vi "Test Trigger VI.vi"() -> ()   [LabVIEW 2011]
uses:
  <vilib>/Utility/file.llb/Write To Spreadsheet File (DBL).vi
panel:
  out "Channel 3 Mean":dbl=1.0
  out "Channel 3 Buffer":dbl[](array[numeric])
  in  "file path (use dialog)":path
  out "V1 Buffer":dbl[](array[numeric]) format="%#_10g"
  out "V1/V2 Buffer":dbl[](array[numeric]) format="%#_10g"
  out "V2 Mean":dbl
  in  "milliseconds to wait":u32=2500
  out "Ratio V1/V2 Mean":dbl=1.0
  out "Shots Measured":ext[][](array[numeric]) format="%#_10g"
  out "V1 Mean":dbl=1.0
  in  "Shots":i32
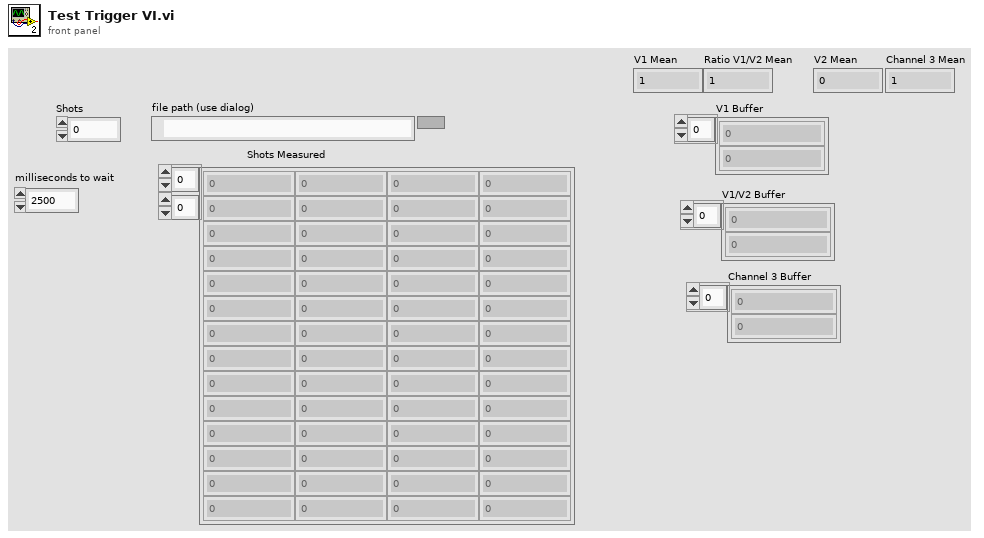
[diagram p1: front panel]
types:
  T1 = enum16{"open", "replace", "create", "open or create", "replace or create", "replace or create with confirmation"}
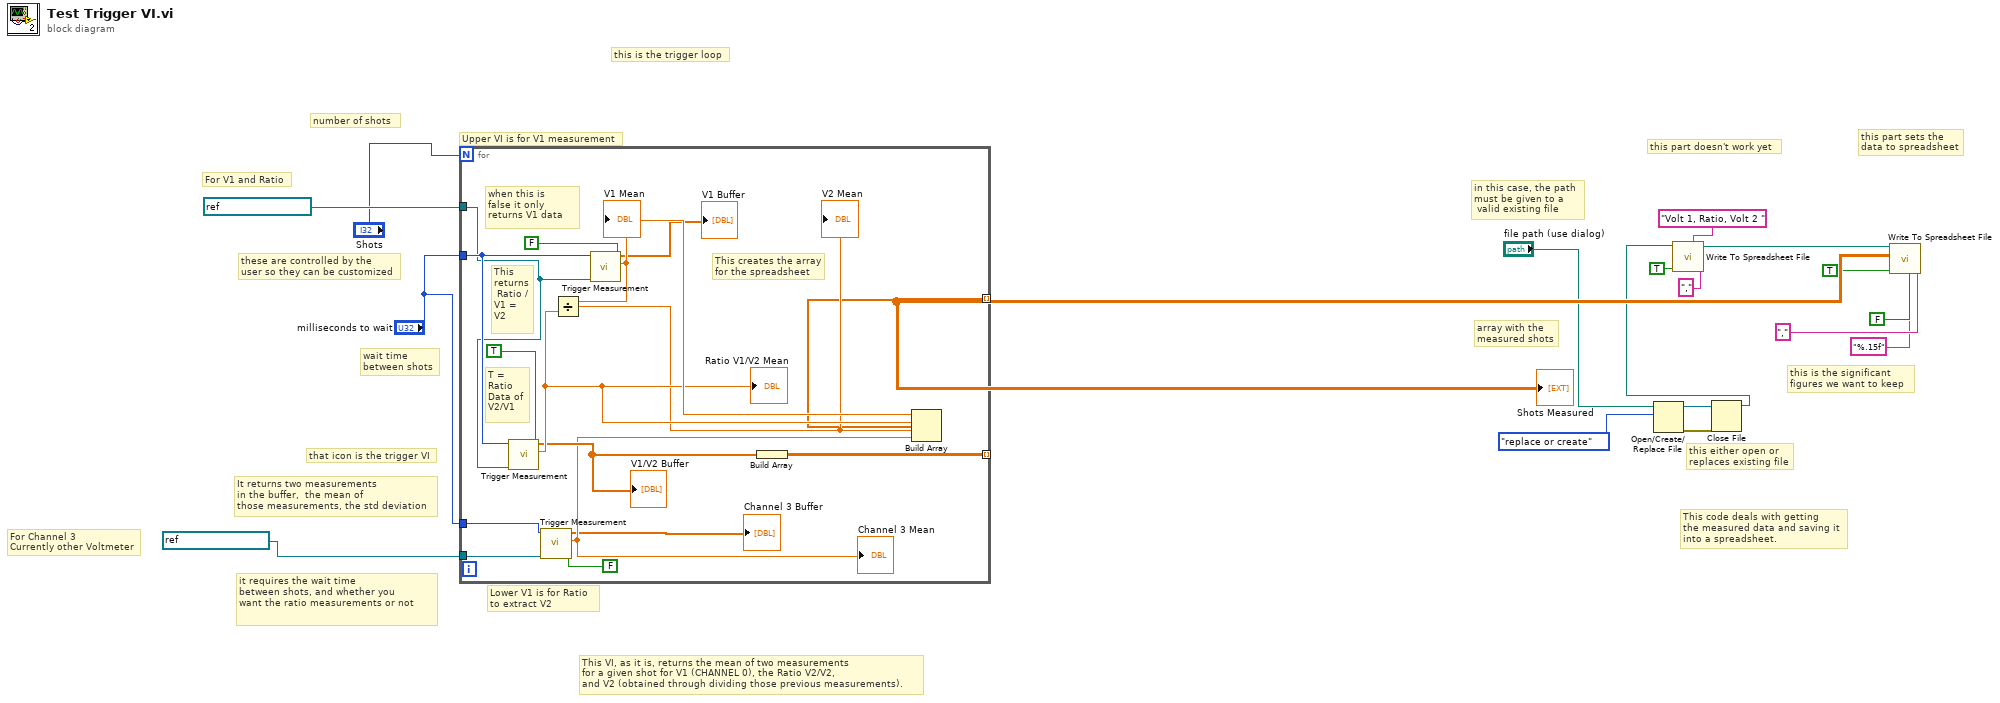
[diagram p0: block diagram]
diagram:
  # "For Channel 3\nCurrently other Voltmeter"
  # "For V1 and Ratio"
  # "This code deals with getting\nthe measured data and saving it\ninto a spreadsheet."
  # "Lower V1 is for Ratio \nto extract V2"
  # "Upper VI is for V1 measurement"
  # "This VI, as it is, returns the mean of two measurements\nfor a given shot for V1 (CHANNEL 0), the Ratio V2/V2, \nand V2 (obtained through dividing those previous measurements)."
  # "it requires the wait time \nbetween shots, and whether you \nwant the ratio measurements or not"
  # "It returns two measurements \nin the buffer,  the mean of \nthose measurements, the std deviation"
  # "that icon is the trigger VI"
  # "this is the trigger loop"
  # "these are controlled by the \nuser so they can be customized"
  # "number of shots"
  # "wait time \nbetween shots"
  # "this is the significant \nfigures we want to keep"
  # "this either open or \nreplaces existing file"
  # "array with the\nmeasured shots"
  # "in this case, the path \nmust be given to a\n valid existing file"
  # "this part sets the \ndata to spreadsheet"
  # "this part doesn't work yet"
  n1 = for {
    N: "Shots" -> [_]
    tunnel: [w27] -> w18 mode=indexing
    tunnel: "milliseconds to wait" -> [w29]
    tunnel: [w25] -> _ mode=indexing
    tunnel: refnum<visa-resource-name> "GPIB0::7::INSTR" ("VISA resource name") -> [w24]
    tunnel: refnum<visa-resource-name> "GPIB0::5::INSTR" ("VISA resource name") -> [w23]
    tunnel: "milliseconds to wait" -> [w22]
    # "This creates the array \nfor the spreadsheet"
    # "T =\nRatio Data of\nV2/V1"
    # "This returns\n Ratio / V1 = V2"
    # "when this is \nfalse it only returns V1 data"
    n2 = call "Trigger Measurement.vi"("Ratio Two Channels \n(Enable V1/V2 Measure)"=TRUE ("Ratio Two Channels \n(Enable V1/V2 Measure)"), "VISA resource name"=w24, "milliseconds to wait"=w29) -> ("Mean"=w31:dbl, "Buffer"=w26:ext[])  [unwired: 6 in, 1 out]
    "Ratio V1/V2 Mean" <- w31
    "V1/V2 Buffer" <- w26
    n3 = call "Trigger Measurement.vi"("Ratio Two Channels \n(Enable V1/V2 Measure)"=FALSE ("Ratio Two Channels \n(Enable V1/V2 Measure)"), "VISA resource name"=w23, "milliseconds to wait"=w22) -> ("Mean"=w20:dbl, "Buffer"=→"Channel 3 Buffer":ext[])  [unwired: 6 in, 1 out]
    "Channel 3 Mean" <- w20
    n4 = call "Trigger Measurement.vi"("Ratio Two Channels \n(Enable V1/V2 Measure)"=FALSE ("Ratio Two Channels \n(Enable V1/V2 Measure)"), "VISA resource name"=w24, "milliseconds to wait"=w29) -> ("Mean"=w32:dbl, "Buffer"=→"V1 Buffer":ext[])  [unwired: 6 in, 1 out]
    "V1 Mean" <- w32
    n5 = Divide(x=w32, y=w31) -> (x/y=w30:dbl)
    "V2 Mean" <- w30
    n6 = Build Array(w26) -> (w25:ext[][])
    n7 = Build Array(w32, w31, w30, w20) -> (w27:dbl[])
  }
  "Shots Measured" <- w18
  n8 = Open/Create/Replace File(file path (use dialog)="file path (use dialog)", operation (0:open)=T1."replace or create") -> (refnum out=w7:refnum<file>, error out=w6:errorcluster)  [unwired: 4 in, 1 out]
  n9 = Close File(refnum=w7, error in=w6) -> (path=w5:path)  [unwired: 1 out]
  n10 = call-poly <vilib>:"Write To Spreadsheet File.vi"("delimiter (\\t)"="," ("delimiter (\\t)"), "format (%.3f)"="Volt 1, Ratio, Volt 2 ", "append to file? (new file:F)"=TRUE, "file path (dialog if empty)"=w5) -> ("new file path (Not A Path if cancelled)"=w10:path)  [unwired: 4 in]
  n11 = call-poly <vilib>:"Write To Spreadsheet File.vi"("delimiter (\\t)"="," ("delimiter (\\t)"), "transpose? (no:F)"=FALSE, "format (%.3f)"="%.15f", "append to file? (new file:F)"=TRUE, "2D data"=w18, "file path (dialog if empty)"=w10) -> ()  [unwired: 2 in, 1 out]
